vi "ChassisDisable.vi"   [LabVIEW 2014, in "ChassisLib.lvlib"]
uses:
  ChassisLib.lvlib
  ChassisRefs.ctl
  <vilib>/Rock Robotics/WPI/RobotDrive/WPI_RobotDriveGetSetRefNum.vi
types:
  T1 = typedef "ChassisLib.lvlib/ChassisRefs.ctl" = enum16{"RobotDrive", "Compressor"}
  T2 = typedef "WPI_CompressorDevRef.ctl" = cluster{"DevStatus":errorcluster, "Pneumatics Control Module":u8}
  T3 = typedef "WPI_RobotDriveDevRef.ctl" = cluster{"DevStatus":errorcluster, "Motors[]":T4[], "Square Inputs":bool, "Max Output":dbl}
  T4 = typedef "WPI_MotorControlDeviceRef.ctl" = cluster{"DeviceStatus":errorcluster, "Type":T5, "PWM":cluster{"Controller":T6, "PWM Channel":T7, "DeadBand":T8}, "CAN":cluster{"Device Number":u8, "Control Mode":T9, "Semaphore":T10, "Max Vout":dbl, "TalonSRX Control Mode":T11}, "Invert":bool, "TransformRef":T12, "InvTransformRef":T12}
  T5 = typedef "WPI_MotorControlType.ctl" = enum16{"PWM", "CAN", "CANTalonSRX"}
  T6 = typedef "FPGA_TypedefDigitalModule.ctl" = enum16{"Controller 1"}
  T7 = typedef "FPGA_DIOPWMChannel.ctl" = enum8{"PWM 0", "PWM 1", "PWM 2", "PWM 3", "PWM 4", "PWM 5", "PWM 6", "PWM 7", "PWM 8", "PWM 9", "PWM MXP 0", "PWM MXP 1", "PWM MXP 2", "PWM MXP 3", "PWM MXP 4", "PWM MXP 5", "PWM MXP 6", "PWM MXP 7", "PWM MXP 8", "PWM MXP 9", "Invalid"}
  T8 = typedef "WPI_PWMDeadband.ctl" = cluster{"Name":string, "maxPositivePwm":i32, "minPositivePwm":i32, "centerPwm":i32, "maxNegativePwm":i32, "minNegativePwm":i32, "angularRange":u16}
  T9 = typedef "WPI_CANJaguar_ControlMode.ctl" = enum8{"Percent VBus", "Current", "Speed", "Position", "Voltage"}
  T10 = typedef "Semaphore RefNum" = refnum<k1>
  T11 = typedef "WPI_CANTalonSRX_APIControlMode.ctl" = enum8{"Percent VBus", "Speed", "Position", "Slave", "Unchanged / Invalid"}
  T12 = typedef "WPI_PWMTransform_ConPane.ctl" = refnum<vi>
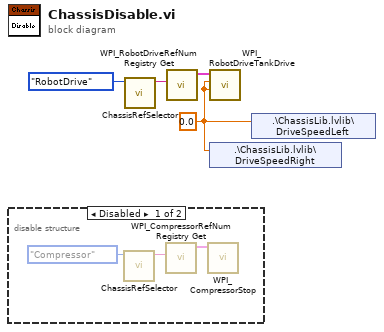
[diagram p0: block diagram]
diagram:
  w1 = 0.0 ("DriveSpeedLeft")
  n1 = disable-structure shown="Disabled" {
    frame Disabled {
      n2 = call "ChassisRefSelector.vi"("Enum 2"=ChassisRefs."Compressor") -> ("String"=w6:string)  [unwired: 10 in]
      n3 = call <vilib>:"WPI_CompressorRefNum Registry Get.vi"("refnum name"=w6) -> ("CompressorDevRef"=w5:T2)  [unwired: 9 in, 1 out]
      n4 = call <vilib>:"WPI_CompressorStop.vi"("CompressorDevRef"=w5) -> ()  [unwired: 9 in, 2 out]
    }
    frame Enabled {
    }
  }
  n5 = call "ChassisRefSelector.vi"("Enum 2"=ChassisRefs."RobotDrive") -> ("String"=w4:string)  [unwired: 10 in]
  n6 = call <vilib>:"WPI_RobotDriveRefNum Registry Get.vi"("refnum name"=w4) -> ("RobotDriveDevRef"=w2:T3)  [unwired: 9 in, 1 out]
  n7 = call <vilib>:"WPI_RobotDriveTankDrive.vi"("Right axis value"=w1, "Left axis value"=w1, "RobotDriveDevRef"=w2) -> ()  [unwired: 6 in, 3 out]
  n8 = shared-variable ".\\ChassisLib.lvlib\\DriveSpeedRight"(w1) -> ()  [unwired: 1 in, 1 out]
  n9 = shared-variable ".\\ChassisLib.lvlib\\DriveSpeedLeft"(w1) -> ()  [unwired: 1 in, 1 out]
